vi "LCR_Main.vi"() -> ()   [LabVIEW 2021]
uses:
  GEN_States.ctl
  1375486a-d526-4950-a4e9-ede105372d37.vi
  Sources/Config_Cluster.ctl
  Sources/Data_Cluster.ctl
  <vilib>/Utility/config.llb/NI_LVConfig.lvlib
  Sources/Mode_Enum.ctl
  Sources/Measurement_Cluster.ctl
  <instrlib>/Hameg HM8118/Hameg HM8118.lvlib
  Sources/Plotting-Axis.ctl
panel:
  in  "Control Tab":enum32{"General", "Configs"}(tab)
  out "Capacitance":dbl
  in  "StopM_Button":bool
  in  "Log_Button":bool
  in  "Measure_Button":bool
  out "Globals":bool
  out "AH 2500A":bool
  out "Logging":bool
  out "Measuring":bool
  out "Magnetic Field":dbl
  out "Temperature":dbl
  in  "LoadConfig_Button":bool
  in  "ApplyConfig_Button":bool
  in  "Measure rate (1/s)":i32
  in  "SaveConfig_Button":bool
  in  "Default Measurement Profile":path
  in  "Retry_Button":bool
  in  "Restart on Load":bool
  in  "Config Path (Blank is default)":path
  in  "LCR VISA COM":refnum<visa-resource-name>
  in  "Global Temp VAR":refnum<k21>
  in  "Global Mag VAR":refnum<k21>
  in  "Logging Path":path
  in  "Display Tab":enum32{"Program Monitor", "Test Plot"}(tab)
  out "Status":string
  in  "Clear_Button":bool
  in  "Y-Axis":T1
  in  "X-Axis":T1
  out "Test Graph":cluster{"X":dbl, "Y":dbl}[](graph)
  in  "Max Elements":i32=5000
  in  "Exit_Button":bool
  # "Instrument Settings"
  # "Global Var. Settings"
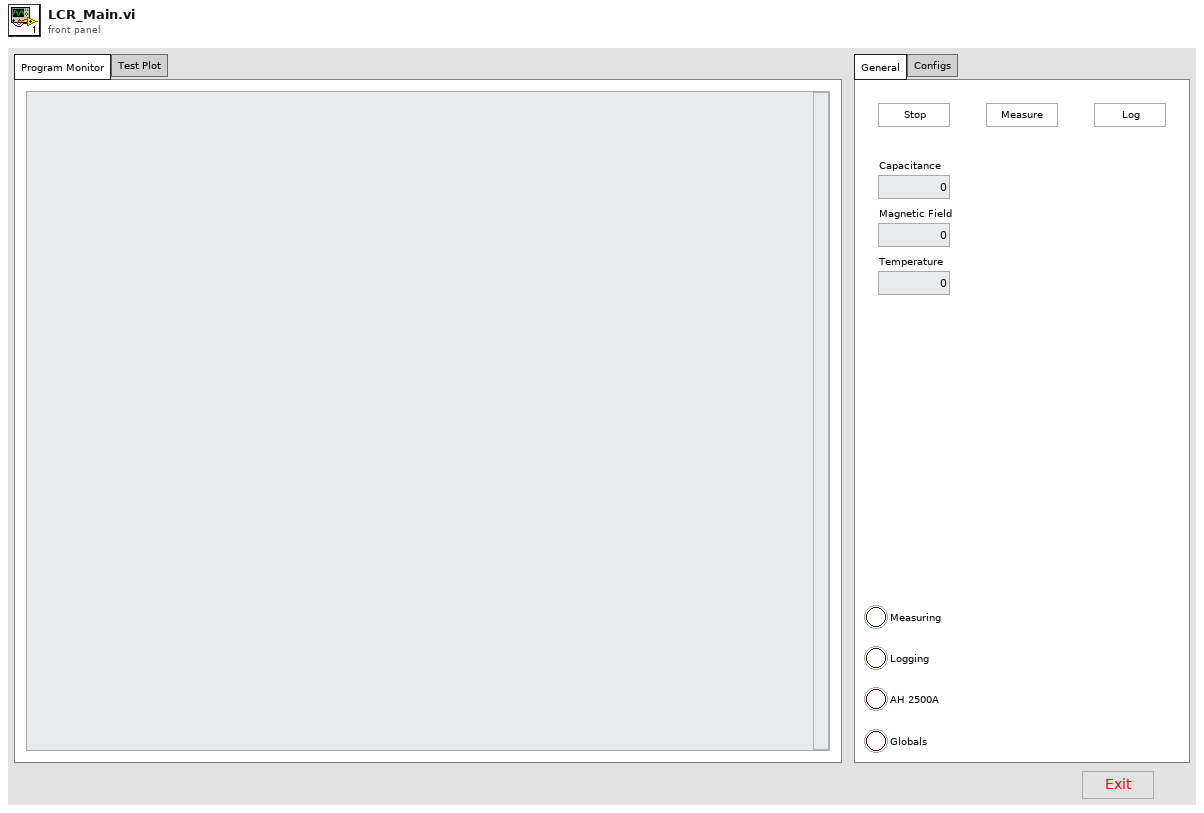
[diagram p1: front panel]
types:
  T1 = typedef "Plotting-Axis.ctl" = enum16{"Time", "Temperature", "MagneticField", "Primary", "Secondary"}
  T2 = typedef "GEN_States.ctl" = enum16{"ClearBuffers", "SwitchToMeas", "SwitchToLog", "SwitchToOff", "Disconnect", "ApplyConfig", "ExitSafe", "RefreshPlotMUnits", "UpdatePlots", "RefreshMUnits", "ChangeOperation", "Read/WriteAll", "RetryComs", "SendProfile", "InitGUI", "RefreshGUI", "ComsFail", "SaveConfig", "Idle", "ProgInit"}
  T3 = typedef "Data_Cluster.ctl" = cluster{"Value":dbl, "GUI Data Cluster":cluster{"Numeric":dbl}, "Timing":cluster{"Last Operation":dbl}, "Measurements":T4[]}
  T4 = typedef "Measurement_Cluster.ctl" = cluster{"Time Stamp":timestamp, "Cap":dbl, "Temperature":dbl, "MagneticField":dbl}
  T5 = typedef "Config_Cluster.ctl" = cluster{"General":cluster{"Config.ini":path, "Default Logging Path":path}, "Hardware":cluster{"AHC VISA COM":refnum<visa-resource-name>, "Measure Rate (1/s)":i32, "Global T VAR":refnum<k21>, "Global B VAR":refnum<k21>}, "Operation":cluster{"Operation Mode":T6, "Status":string, "NewLog?":bool}}
  T6 = typedef "Mode_Enum.ctl" = enum16{"Logging", "Idle-Off", "Idle"}
  T7 = enum8{"Enabled", "Disabled", "Disabled and Grayed Out"}
  T8 = typedef "NI_LVConfig.lvlib/Config Data RefNum.ctl" = refnum<k1>
  T9 = cluster{"Logging Path":path, "LCR VISA COM":refnum<visa-resource-name>, "Restart on Load":bool, "Default Measurement Profile":path, "Measure rate (1/s)":i32, "Global Temp VAR":refnum<k21>, "Global Mag VAR":refnum<k21>}
  T10 = cluster{"Primary Measurement":dbl, "Secondary Measurement":dbl, "T Var":dbl, "B Var":dbl}
  T11 = typedef "UnitEnum.ctl" = enum16{"L", "R", "C", "Z", "X", "Q", "Theta", "Y", "N", "M", "G", "B", "D"}
  T12 = typedef "GEN_States.ctl" = enum16{"ClearBuffers", "SwitchToMeas", "SwitchToLog", "SwitchToOff", "Disconnect", "ApplyConfig", "ExitSafe", "RefreshPlotMUnits", "UpdatePlots", "RefreshMUnits", "ChangeOperation", "Read/WriteAll", "RetryComs", "SendProfile", "InitGUI", "RefreshGUI", "ComsFail", "LoadProfile", "SaveProfile", "SaveConfig", "Idle", "ProgInit"}
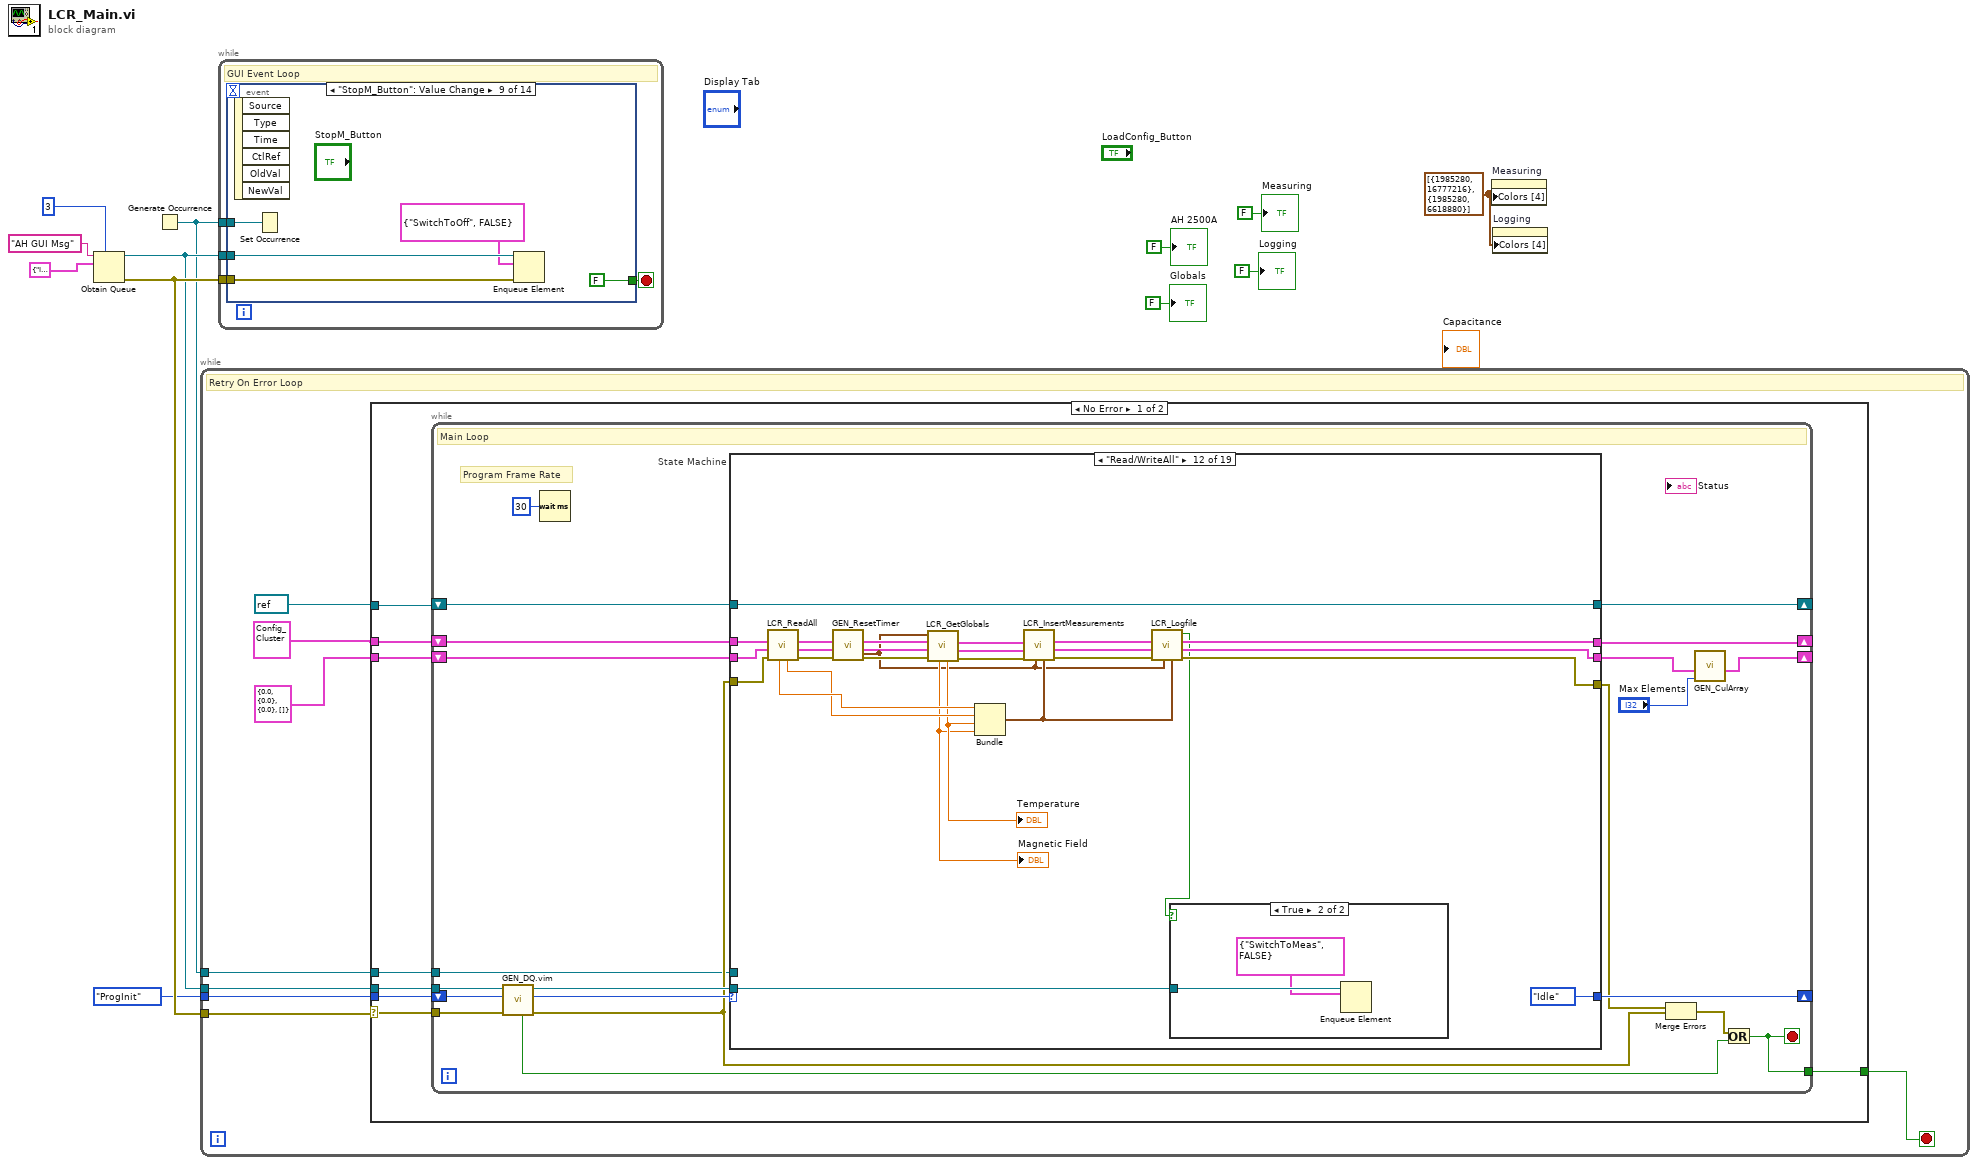
[diagram p0: block diagram]
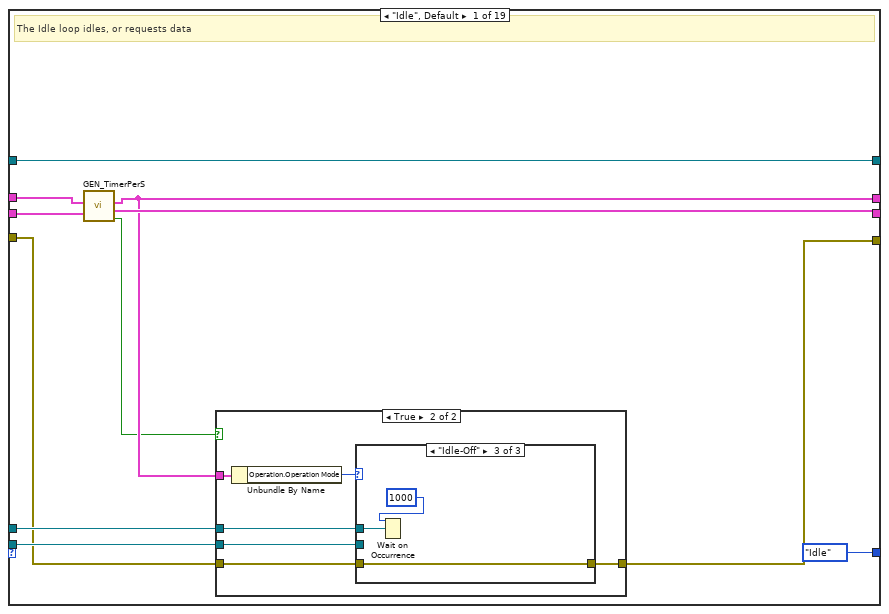
[diagram p2: hidden frame]
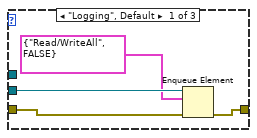
[diagram p4: hidden frame]
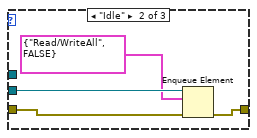
[diagram p5: hidden frame]
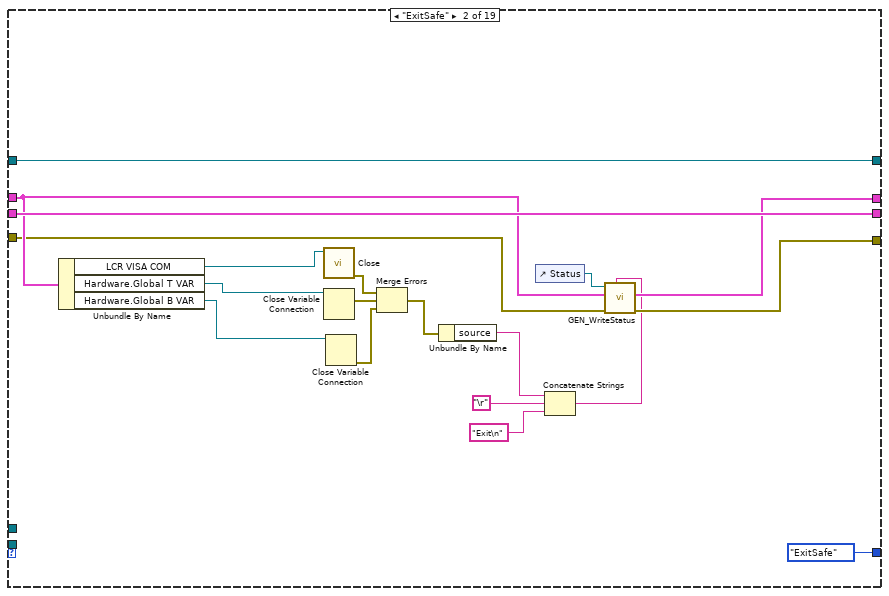
[diagram p6: hidden frame]
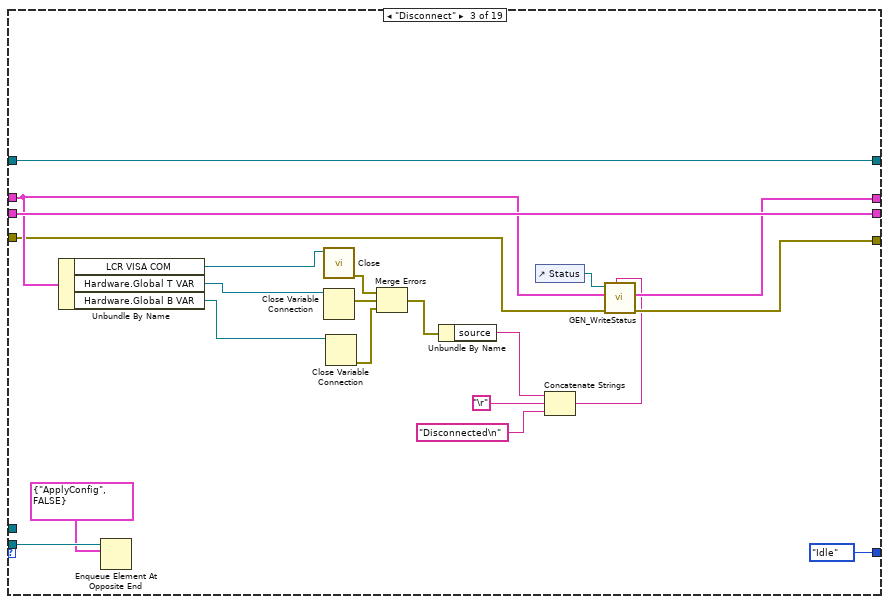
[diagram p7: hidden frame]
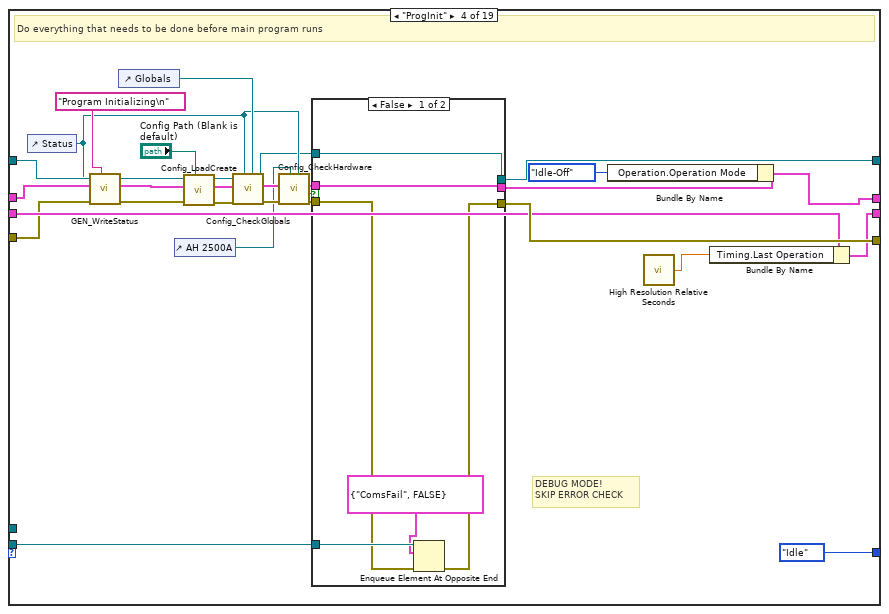
[diagram p8: hidden frame]
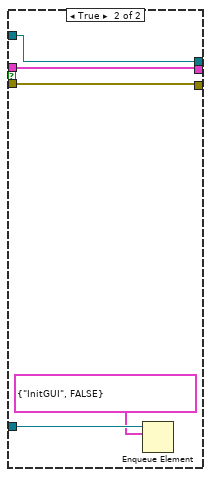
[diagram p9: hidden frame]
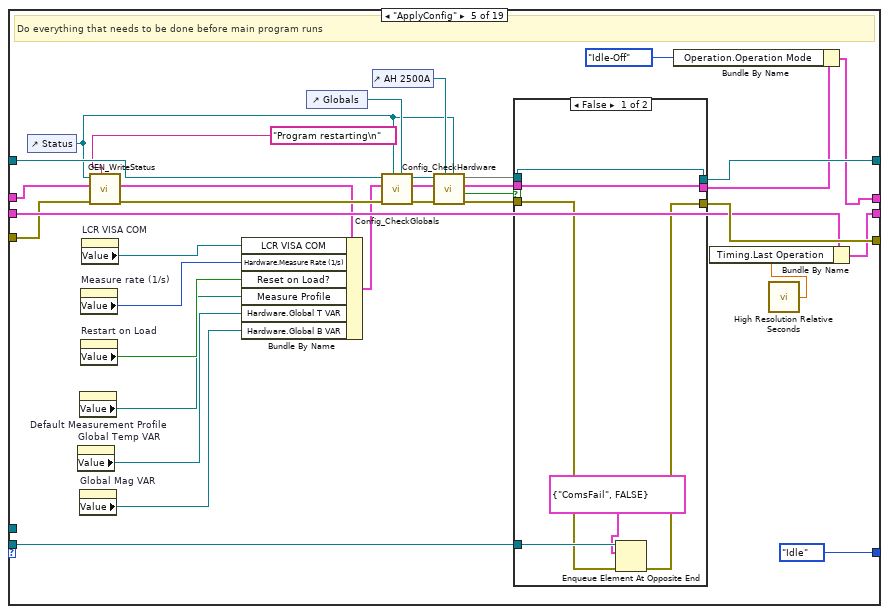
[diagram p10: hidden frame]
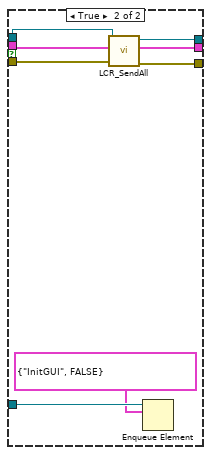
[diagram p11: hidden frame]
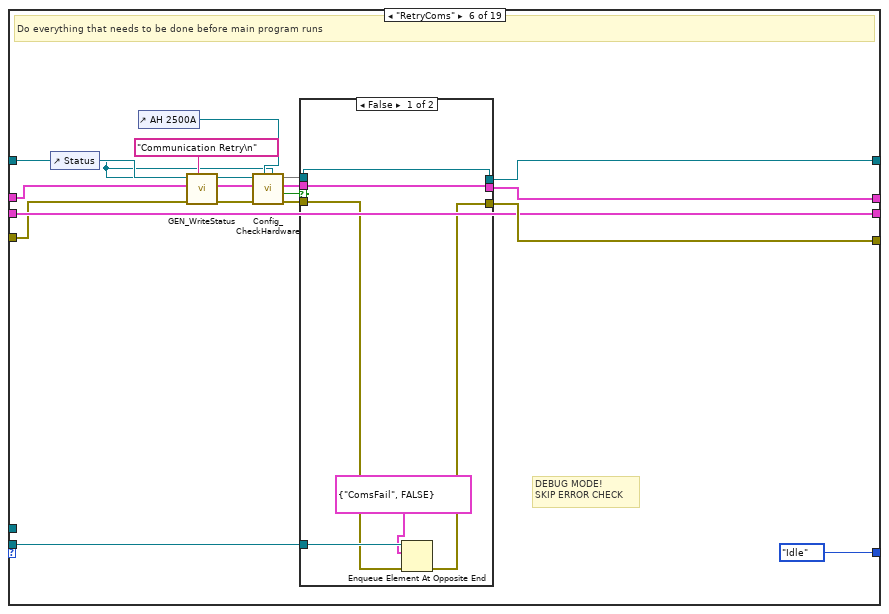
[diagram p12: hidden frame]
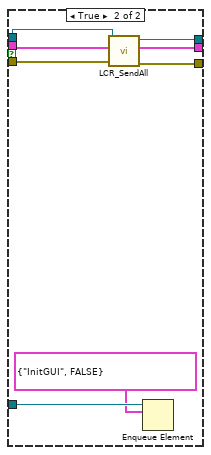
[diagram p13: hidden frame]
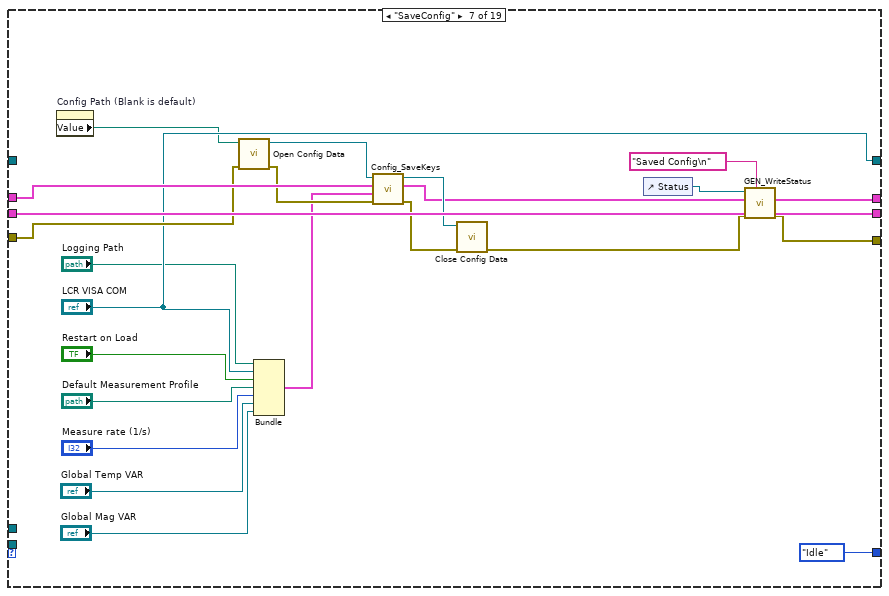
[diagram p14: hidden frame]
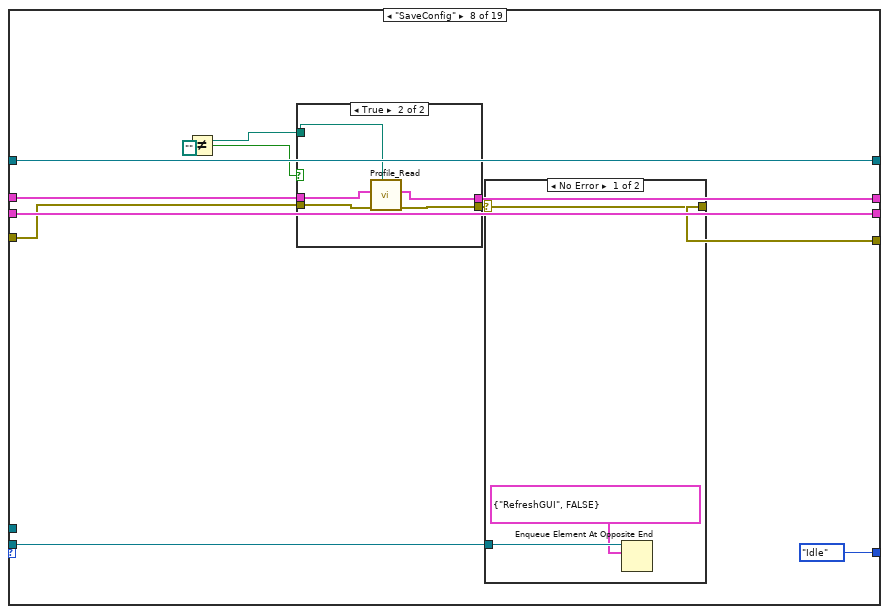
[diagram p15: hidden frame]
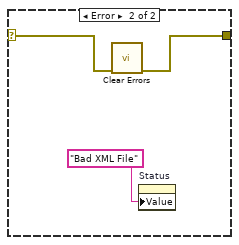
[diagram p16: hidden frame]
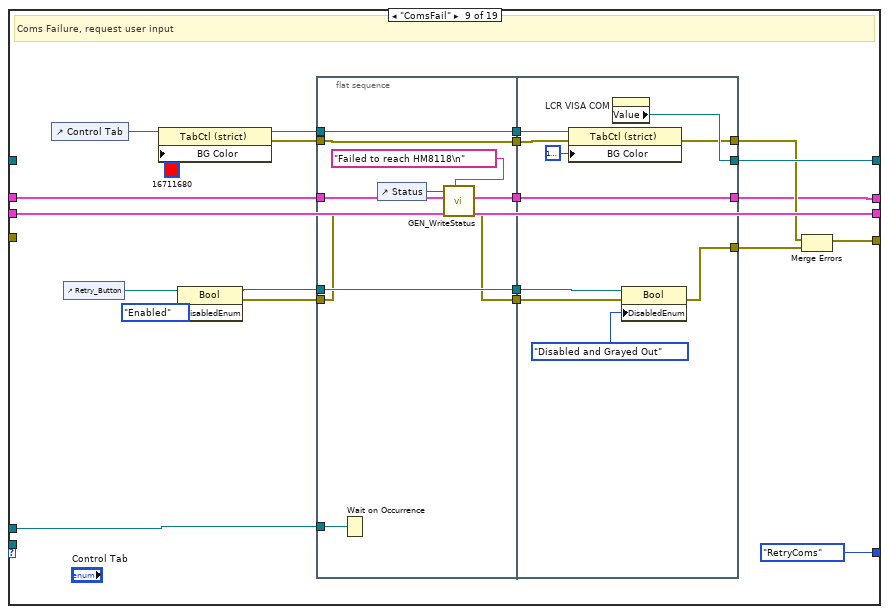
[diagram p18: hidden frame]
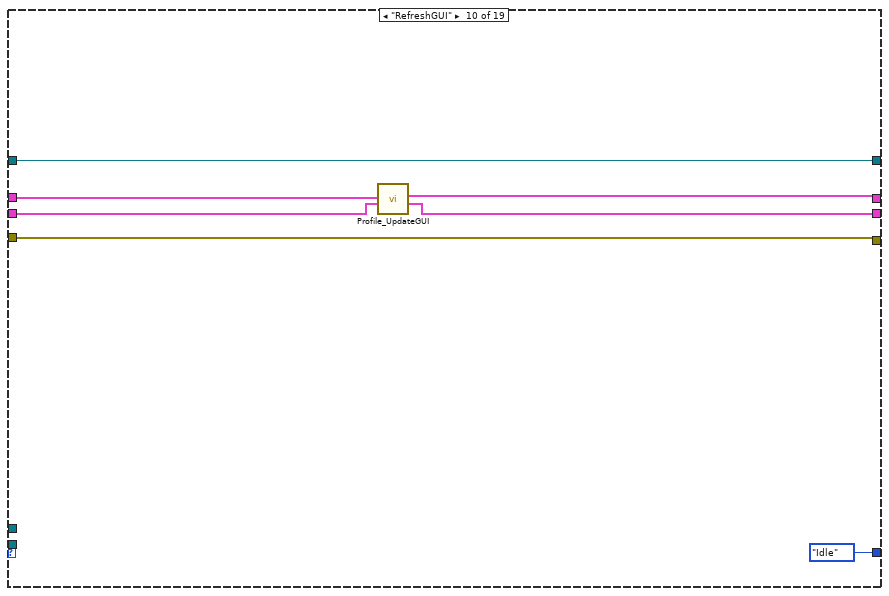
[diagram p19: hidden frame]
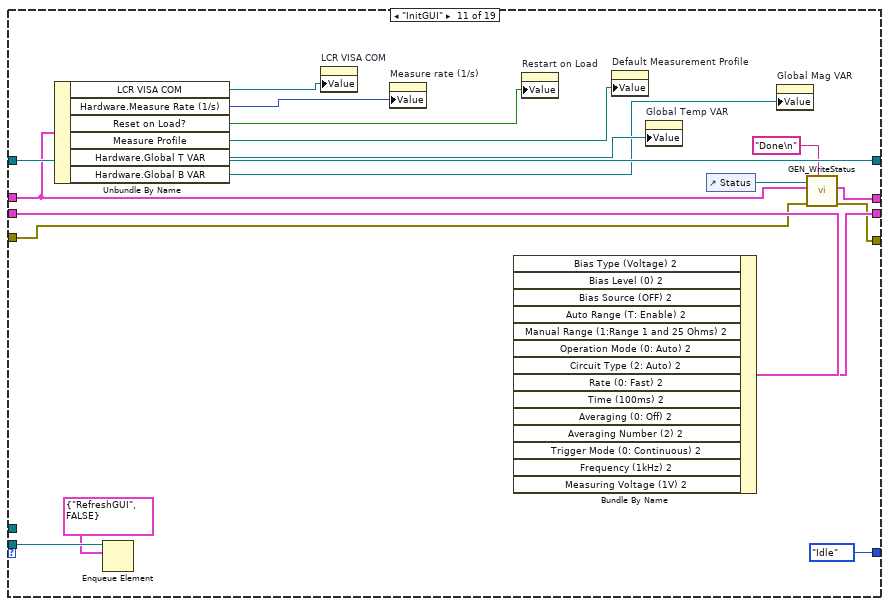
[diagram p20: hidden frame]
diagram:
  w1 = cluster{u32, u32}[] [{1985280, 16777216}, {1985280, 6618880}] ("Colors [4]")
  n1 = Obtain Queue(max queue size (-1, unlimited)=3, name (unnamed)="AH GUI Msg", element data type=cluster{T2, bool} {enum."Idle", TRUE}) -> (queue out=w8:refnum<queue>, error out=w9:errorcluster)  [unwired: 2 in, 1 out]
  n2 = Generate Occurrence() -> (w6:refnum<k4>)
  n3 = while {
    tunnel: w9 -> [w20]
    tunnel: w8 -> [w19]
    tunnel: GEN_States."ProgInit" ("State") -> [w18]
    tunnel: w6 -> [w13]
    stop <- w17 stop-if-true
    # "Retry On Error Loop"
    n4 = case shown="No Error" w20 {
      selector: w20 -> [w28 _]
      tunnel: w19 -> [w27 _]
      tunnel: w18 -> [w26 _]
      tunnel: [w25 TRUE] -> w17
      tunnel: refnum<visa-resource-name> refnum ("LCR VISA COM") -> [w24 _]
      tunnel: T5 {"General"={"Config.ini"=path "", "Default Logging Path"=path ""}, "Hardware"={"AHC VISA COM"="", "Measure Rate (1/s)"=0, "Global T VAR"="", "Global B VAR"=""}, "Operation"={"Operation Mode"=enum."Logging", "Status"="", "NewLog?"=FALSE}} -> [w23 _]
      tunnel: T3 {"Value"=0.0, "GUI Data Cluster"={"Numeric"=0.0}, "Timing"={"Last Operation"=0.0}, "Measurements"=[]} -> [w22 _]
      tunnel: w13 -> [w21 _]
      frame No Error {
        n5 = while {
          tunnel: w28 -> [w48]
          tunnel: w27 -> [w47]
          shift-right: [w40] -> _
          shift-left: w26 -> [w46]
          tunnel: [w42] -> w25
          shift-right: [w39] -> _
          shift-left: w24 -> [w41]
          shift-right: [w36] -> _
          shift-left: w23 -> [w37]
          shift-right: [w30] -> _
          shift-left: w22 -> [w35]
          tunnel: w21 -> [w32]
          stop <- w42 stop-if-true
          # "Program Frame Rate"
          # "Main Loop"
          n6 = call "GEN_DQ.vim"("error in (no error)"=w48, "Variant"=w46, "queue In"=w47) -> ("error out"=w34:errorcluster, "Variant Out"=w45:T2, "queue out"=w38:refnum<queue>, "Exit?"=w43:bool)  [unwired: 5 in]
          n7 = Wait (ms)(milliseconds to wait=u32 30) -> ()  [unwired: 1 out]
          n8 = case "State Machine" shown="\"Read/WriteAll\"" w45 {
            tunnel: w41 -> [w60 w97 w118 w145 w190 w222 _ w272 _ w333 w366 w394 w413 w431 w457 w476 w487 w497 w503]
            tunnel: [GEN_States."Idle" ("State") GEN_States."ExitSafe" ("State") GEN_States."Idle" ("State") GEN_States."Idle" ("State") GEN_States."Idle" ("State") GEN_States."Idle" ("State") GEN_States."Idle" ("State") GEN_States."Idle" ("State") GEN_States."RetryComs" ("State") GEN_States."Idle" ("State") GEN_States."Idle" ("State") GEN_States."Idle" ("State") GEN_States."Idle" ("State") GEN_States."Idle" ("State") w443 GEN_States."Idle" ("State") GEN_States."Idle" ("State") GEN_States."Idle" ("State") GEN_States."Idle" ("State")] -> w40
            tunnel: [w60 w97 w118 w140 w184 w215 "LCR VISA COM" w272 w300 w333 w366 w394 w413 w431 w457 w476 w487 w497 w503] -> w39
            tunnel: w38 -> [w57 _ w100 w139 w183 w214 _ w261 _ _ w362 w367 _ _ _ _ _ _ _]
            tunnel: w37 -> [w54 w90 w112 w131 w175 w212 w255 w268 w288 w328 w342 w393 w411 w429 w455 w477 w486 w494 w502]
            tunnel: [w51 w89 w111 w132 w176 w216 w245 w267 w287 w330 w341 w388 w408 w426 w444 w474 w486 w494 w502] -> w36
            tunnel: w35 -> [w53 w96 w117 w138 w182 w213 w260 w271 w302 w331 w365 w385 w412 w430 w456 w475 w482 w495 w500]
            tunnel: [w52 w96 w117 w137 w181 w213 w260 w271 w302 w329 w364 w382 w412 w430 w456 w475 w481 w495 w499] -> w31
            tunnel: w34 -> [w56 w88 w110 w129 w174 w209 w254 w269 _ w332 w339 w392 w403 w421 w449 w473 w480 w493 w501]
            tunnel: [w55 w87 w109 w141 w185 w217 w241 w262 w291 w332 w338 w389 w402 w420 w448 w468 w480 w493 w501] -> w33
            tunnel: w32 -> [w58 _ _ _ _ _ _ _ w301 _ _ _ _ _ _ _ _ _ _]
            frame "Idle", Default {
              # "The Idle loop idles, or requests data"
              n9 = call "GEN_TimerPerS.vi"("Data_In"=w53, "Config_In"=w54) -> ("Time"=w50:bool, "Data_In 2"=w52:T3, "Config_In 2"=w51:T5)  [unwired: 7 in]
              n10 = case shown="True" w50 {
                tunnel: w58 -> [_ w66]
                tunnel: w57 -> [_ w65]
                tunnel: w56 -> [w61 w64]
                tunnel: [w61 w63] -> w55
                tunnel: w51 -> [_ w62]
                frame False {
                }
                frame True {
                  n11 = Unbundle By Name(w62) -> ("Operation.Operation Mode"=w67:T6)
                  n12 = case shown="\"Idle-Off\"" w67 {
                    tunnel: w66 -> [_ _ w78]
                    tunnel: w65 -> [w71 w75 _]
                    tunnel: w64 -> [w70 w74 w77]
                    tunnel: [w68 w72 w77] -> w63
                    frame "Logging", Default {
                      n13 = Enqueue Element(queue=w71, element=cluster{T2, bool} {enum."Read/WriteAll", FALSE}, error in (no error)=w70) -> (error out=w68:errorcluster)  [unwired: 1 in, 2 out]
                    }
                    frame "Idle" {
                      n14 = Enqueue Element(queue=w75, element=cluster{T2, bool} {enum."Read/WriteAll", FALSE}, error in (no error)=w74) -> (error out=w72:errorcluster)  [unwired: 1 in, 2 out]
                    }
                    frame "Idle-Off" {
                      n15 = Wait on Occurrence(2:w78, 3:1000 ("ms timeout (-1)")) -> ()  [unwired: 1 in, 1 out]
                    }
                  }
                }
              }
            }
            frame "ExitSafe" {
              n16 = Unbundle By Name(w90) -> ("LCR VISA COM"=w94:refnum<visa-resource-name>, "Hardware.Global T VAR"=w93:refnum<k21>, "Hardware.Global B VAR"=w92:refnum<k21>)
              n17 = call <instrlib>:"Close.vi"("VISA resource name"=w94) -> ("error out"=w84:errorcluster)  [unwired: 10 in]
              n18 = Close Variable Connection(11:w93) -> (0:w85:errorcluster)  [unwired: 1 in]
              n19 = Close Variable Connection(11:w92) -> (0:w86:errorcluster)  [unwired: 1 in]
              n20 = Merge Errors(w84, w85, w86) -> (w83:errorcluster)
              n21 = Unbundle By Name(w83) -> ("source"=w81:string)
              n22 = control-ref of="Status"() -> (w91:refnum<vi>)
              n23 = Concatenate Strings(w81, "\r", "Exit\n" ("string")) -> (w82:string)
              n24 = call "GEN_WriteStatus.vi"("Input String"=w82, "error in (no error)"=w88, "Config_Cluster"=w90, "Status Ref"=w91) -> ("error out"=w87:errorcluster, "Config_Cluster Out"=w89:T5)  [unwired: 6 in]
            }
            frame "Disconnect" {
              n25 = Unbundle By Name(w112) -> ("LCR VISA COM"=w116:refnum<visa-resource-name>, "Hardware.Global T VAR"=w115:refnum<k21>, "Hardware.Global B VAR"=w114:refnum<k21>)
              n26 = Enqueue Element At Opposite End(queue=w100, element=cluster{T2, bool} {enum."ApplyConfig", FALSE}) -> ()  [unwired: 2 in, 3 out]
              n27 = call <instrlib>:"Close.vi"("VISA resource name"=w116) -> ("error out"=w106:errorcluster)  [unwired: 10 in]
              n28 = Close Variable Connection(11:w115) -> (0:w107:errorcluster)  [unwired: 1 in]
              n29 = Close Variable Connection(11:w114) -> (0:w108:errorcluster)  [unwired: 1 in]
              n30 = Merge Errors(w106, w107, w108) -> (w105:errorcluster)
              n31 = Unbundle By Name(w105) -> ("source"=w103:string)
              n32 = control-ref of="Status"() -> (w113:refnum<vi>)
              n33 = Concatenate Strings(w103, "\r", "Disconnected\n" ("string")) -> (w104:string)
              n34 = call "GEN_WriteStatus.vi"("Input String"=w104, "error in (no error)"=w110, "Config_Cluster"=w112, "Status Ref"=w113) -> ("error out"=w109:errorcluster, "Config_Cluster Out"=w111:T5)  [unwired: 6 in]
            }
            frame "ProgInit" {
              # "DEBUG MODE!\nSKIP ERROR CHECK"
              # "Do everything that needs to be done before main program runs"
              n35 = control-ref of="Status"() -> (w120:refnum<vi>)
              n36 = call "GEN_WriteStatus.vi"("Input String"="Program Initializing\n" ("Status"), "error in (no error)"=w129, "Config_Cluster"=w131, "Status Ref"=w120) -> ("error out"=w128:errorcluster, "Config_Cluster Out"=w130:T5)  [unwired: 6 in]
              n37 = control-ref of="Globals"() -> (w122:refnum<vi>)
              n38 = control-ref of="AH 2500A"() -> (w121:refnum<vi>)
              n39 = call "Config_LoadCreate.vi"("Config In"="Config Path (Blank is default)", "error In"=w128, "Configuration Cluster"=w130, "AH VISA COM"=w145) -> ("error out"=w124:errorcluster, "Configuration Cluster Out"=w125:T5, "AHC VISA COM Out"=w127:refnum<visa-resource-name>)  [unwired: 5 in]
              n40 = call "Config_CheckGlobals.vi"("GlobalsLED Ref"=w122, "Status Ref"=w120, "error in (no error)"=w124, "Config Cluster"=w125, "VISA resource name"=w127) -> ("error out"=w123:errorcluster, "Config Cluster Out"=w126:T5, "VISA resource name out"=w119:refnum<visa-resource-name>)  [unwired: 4 in]
              n41 = call "Config_CheckHardware.vi"("Status Ref"=w120, "HM 8119"=w121, "error in (no error)"=w123, "Config Cluster"=w126) -> ("error out"=w143:errorcluster, "Connected?"=w144:bool, "Config Cluster Out"=w142:T5)  [unwired: 5 in]
              n42 = case shown="False" w144 {
                tunnel: w143 -> [w149 w157]
                tunnel: w142 -> [w152 w158]
                tunnel: w119 -> [w153 w154]
                tunnel: [w153 w154] -> w140
                tunnel: [w152 w158] -> w135
                tunnel: [w148 w157] -> w141
                tunnel: w139 -> [w151 w156]
                frame False {
                  n43 = Enqueue Element At Opposite End(queue=w151, element=cluster{T2, bool} {enum."ComsFail", FALSE}, error in (no error)=w149) -> (error out=w148:errorcluster)  [unwired: 1 in, 2 out]
                }
                frame True {
                  n44 = Enqueue Element(queue=w156, element=cluster{T2, bool} {enum."InitGUI", FALSE}) -> ()  [unwired: 2 in, 3 out]
                }
              }
              n45 = Bundle By Name(cluster=w135, "Operation.Operation Mode"=Mode_Enum."Idle-Off") -> (w132:T5)
              n46 = call <vilib>:"High Resolution Relative Seconds.vi"() -> ("relative seconds"=w136:dbl)
              n47 = Bundle By Name(cluster=w138, "Timing.Last Operation"=w136) -> (w137:T3)
            }
            frame "ApplyConfig" {
              # "Do everything that needs to be done before main program runs"
              n48 = control-ref of="Status"() -> (w159:refnum<vi>)
              n49 = property on="Global Temp VAR" class="Variable (strict)"() -> ("Value"=w163:refnum<k21>)  [unwired: 2 in, 2 out]
              n50 = property on="Default Measurement Profile" class="Path"() -> ("Value"=w164:path)  [unwired: 2 in, 2 out]
              n51 = property on="Global Mag VAR" class="Variable (strict)"() -> ("Value"=w162:refnum<k21>)  [unwired: 2 in, 2 out]
              n52 = property on="Measure rate (1/s)" class="DigNum (strict)"() -> ("Value"=w166:i32)  [unwired: 2 in, 2 out]
              n53 = property on="Restart on Load" class="Bool (strict)"() -> ("Value"=w165:bool)  [unwired: 2 in, 2 out]
              n54 = property on="LCR VISA COM" class="VISAName"() -> ("Value"=w167:refnum<visa-resource-name>)  [unwired: 2 in, 2 out]
              n55 = call "GEN_WriteStatus.vi"("Input String"="Program restarting\n" ("Status"), "error in (no error)"=w174, "Config_Cluster"=w175, "Status Ref"=w159) -> ("error out"=w173:errorcluster, "Config_Cluster Out"=w169:T5)  [unwired: 6 in]
              n56 = Bundle By Name(cluster=w169, "LCR VISA COM"=w167, "Hardware.Measure Rate (1/s)"=w166, "Reset on Load?"=w165, "Measure Profile"=w164, "Hardware.Global T VAR"=w163, "Hardware.Global B VAR"=w162) -> (w168:T5)
              n57 = control-ref of="Globals"() -> (w161:refnum<vi>)
              n58 = control-ref of="AH 2500A"() -> (w160:refnum<vi>)
              n59 = call "Config_CheckGlobals.vi"("GlobalsLED Ref"=w161, "Status Ref"=w159, "error in (no error)"=w173, "Config Cluster"=w168, "VISA resource name"=w190) -> ("error out"=w170:errorcluster, "Config Cluster Out"=w171:T5, "VISA resource name out"=w172:refnum<visa-resource-name>)  [unwired: 4 in]
              n60 = call "Config_CheckHardware.vi"("Status Ref"=w159, "HM 8119"=w160, "error in (no error)"=w170, "Config Cluster"=w171, 11:w172) -> ("error out"=w188:errorcluster, "Connected?"=w189:bool, "Config Cluster Out"=w187:T5, 3:w186)  [unwired: 3 in]
              n61 = case shown="False" w189 {
                tunnel: w188 -> [w193 w203]
                tunnel: w187 -> [w196 w204]
                tunnel: w186 -> [w197 w205]
                tunnel: [w197 w202] -> w184
                tunnel: [w196 w201] -> w179
                tunnel: [w192 w200] -> w185
                tunnel: w183 -> [w195 w199]
                frame False {
                  n62 = Enqueue Element At Opposite End(queue=w195, element=cluster{T2, bool} {enum."ComsFail", FALSE}, error in (no error)=w193) -> (error out=w192:errorcluster)  [unwired: 1 in, 2 out]
                }
                frame True {
                  n63 = call "LCR_SendAll.vi"("error in (no error)"=w203, "Configuration Cluster"=w204, "VISA resource name"=w205) -> ("error out"=w200:errorcluster, "Configuration Cluster Out"=w201:T5, "VISA resource name out"=w202:refnum<visa-resource-name>)  [unwired: 6 in]
                  n64 = Enqueue Element(queue=w199, element=cluster{T2, bool} {enum."InitGUI", FALSE}) -> ()  [unwired: 2 in, 3 out]
                }
              }
              n65 = Bundle By Name(cluster=w179, "Operation.Operation Mode"=Mode_Enum."Idle-Off") -> (w176:T5)
              n66 = call <vilib>:"High Resolution Relative Seconds.vi"() -> ("relative seconds"=w180:dbl)
              n67 = Bundle By Name(cluster=w182, "Timing.Last Operation"=w180) -> (w181:T3)
            }
            frame "RetryComs" {
              # "DEBUG MODE!\nSKIP ERROR CHECK"
              # "Do everything that needs to be done before main program runs"
              n68 = control-ref of="Status"() -> (w206:refnum<vi>)
              n69 = control-ref of="AH 2500A"() -> (w207:refnum<vi>)
              n70 = call "GEN_WriteStatus.vi"("Input String"="Communication Retry\n", "error in (no error)"=w209, "Config_Cluster"=w212, "Status Ref"=w206) -> ("error out"=w208:errorcluster, "Config_Cluster Out"=w211:T5)  [unwired: 6 in]
              n71 = call "Config_CheckHardware.vi"("Status Ref"=w206, "HM 8119"=w207, "error in (no error)"=w208, "Config Cluster"=w211, 11:w222) -> ("error out"=w220:errorcluster, "Connected?"=w221:bool, "Config Cluster Out"=w219:T5, 3:w218)  [unwired: 3 in]
              n72 = case shown="False" w221 {
                tunnel: w220 -> [w225 w235]
                tunnel: w219 -> [w228 w236]
                tunnel: w218 -> [w229 w237]
                tunnel: [w229 w234] -> w215
                tunnel: [w228 w233] -> w216
                tunnel: [w224 w232] -> w217
                tunnel: w214 -> [w227 w231]
                frame False {
                  n73 = Enqueue Element At Opposite End(queue=w227, element=cluster{T2, bool} {enum."ComsFail", FALSE}, error in (no error)=w225) -> (error out=w224:errorcluster)  [unwired: 1 in, 2 out]
                }
                frame True {
                  n74 = call "LCR_SendAll.vi"("error in (no error)"=w235, "Configuration Cluster"=w236, "VISA resource name"=w237) -> ("error out"=w232:errorcluster, "Configuration Cluster Out"=w233:T5, "VISA resource name out"=w234:refnum<visa-resource-name>)  [unwired: 6 in]
                  n75 = Enqueue Element(queue=w231, element=cluster{T2, bool} {enum."InitGUI", FALSE}) -> ()  [unwired: 2 in, 3 out]
                }
              }
            }
            frame "SaveConfig" {
              n76 = property on="Config Path (Blank is default)" class="Path"() -> ("Value"=w248:path)  [unwired: 2 in, 2 out]
              n77 = call <vilib>:"Open Config Data.vi"("error in (no error)"=w254, "configuration file path"=w248) -> ("error out"=w253:errorcluster, "refnum"=w252:T8)  [unwired: 7 in, 1 out]
              n78 = Bundle("Logging Path"="Logging Path", "LCR VISA COM"="LCR VISA COM", "Restart on Load"="Restart on Load", "Default Measurement Profile"="Default Measurement Profile", "Measure rate (1/s)"="Measure rate (1/s)", "Global Temp VAR"="Global Temp VAR", "Global Mag VAR"="Global Mag VAR") -> (w238:T9)  [unwired: 1 in]
              n79 = call "Config_SaveKeys.vi"("error in (no error)"=w253, "Settings In"=w238, "Configuration Cluster"=w255, "Config In"=w252) -> ("error out"=w250:errorcluster, "output cluster"=w246:T5, "refnum out"=w251:T8)  [unwired: 5 in]
              n80 = call <vilib>:"Close Config Data.vi"("error in (no error)"=w250, "refnum"=w251) -> ("error out"=w242:errorcluster)  [unwired: 8 in, 1 out]
              n81 = control-ref of="Status"() -> (w243:refnum<vi>)
              n82 = call "GEN_WriteStatus.vi"("Input String"="Saved Config\n", "error in (no error)"=w242, "Config_Cluster"=w246, "Status Ref"=w243) -> ("error out"=w241:errorcluster, "Config_Cluster Out"=w245:T5)  [unwired: 6 in]
            }
            frame "SaveConfig" {
              n83 = Not Equal?(x=w266, y=path "") -> (x != y?=w264:bool)
              n84 = case shown="True" w264 {
                tunnel: w269 -> [w279 w285]
                tunnel: w268 -> [w280 w284]
                tunnel: [_ w283] -> w266
                tunnel: [w279 w282] -> w263
                tunnel: [w280 w281] -> w267
                frame False {
                }
                frame True {
                  n85 = call "Profile_Read.vi"("Measurement Profile"=w283, "error in (no error)"=w285, "Configuration Cluster"=w284) -> ("error out"=w282:errorcluster, "Configuration Cluster Out"=w281:T5)  [unwired: 7 in]
                }
              }
              n86 = case shown="No Error" w263 {
                selector: w263 -> [w275 w278]
                tunnel: [w275 w277] -> w262
                tunnel: w261 -> [w274 _]
                frame No Error {
                  n87 = Enqueue Element At Opposite End(queue=w274, element=cluster{T2, bool} {enum."RefreshGUI", FALSE}) -> ()  [unwired: 2 in, 3 out]
                }
                frame Error {
                  n88 = call <vilib>:"Clear Errors.vi"("error in (no error)"=w278) -> ("error out"=w277:errorcluster)  [unwired: 5 in, 1 out]
                  n89 = property on="Status" class="Str"("Value"="Bad XML File" ("Status")) -> ()  [unwired: 2 in, 2 out]
                }
              }
            }
            frame "ComsFail" {
              # "Coms Failure, request user input"
              n90 = control-ref of="Control Tab"() -> (w307:refnum<vi>)
              n91 = control-ref of="Retry_Button"() -> (w306:refnum<vi>)
              n92 = property on="Property Node" class="TabCtl (strict)"(reference=w307, "BG Color"=u32 16711680 ("Colors:BG Color")) -> (reference out=w298:refnum<vi>, error out=w297:errorcluster)  [unwired: 1 in]
              n93 = property class="Bool"(reference=w306, "DisabledEnum"=T7."Enabled" ("Disabled")) -> (reference out=w294:refnum<vi>, error out=w293:errorcluster)  [unwired: 1 in]
              n94 = flat-sequence {
                tunnel: w301 -> [w317]
                tunnel: [w316] -> w299
                tunnel: w298 -> [w316]
                tunnel: w297 -> [w315]
                tunnel: [w315] -> w296
                tunnel: [w314] -> w295
                tunnel: w294 -> [w314]
                tunnel: w293 -> [w310]
                tunnel: [w309] -> w292
                tunnel: w288 -> [w313]
                tunnel: [w312] -> w286
                tunnel: [w327] -> w300
                tunnel: w299 -> [w326]
                tunnel: w296 -> [w325]
                tunnel: w295 -> [w324]
                tunnel: w292 -> [w323]
                tunnel: [w321] -> w290
                tunnel: [w320] -> w289
                tunnel: [w318] -> w287
                tunnel: w286 -> [w318]
                frame #0 {
                  n95 = Wait on Occurrence(2:w317) -> ()  [unwired: 2 in, 1 out]
                  n96 = control-ref of="Status"() -> (w308:refnum<vi>)
                  n97 = call "GEN_WriteStatus.vi"("Input String"="Failed to reach HM8118\n", "error in (no error)"=w310, "Config_Cluster"=w313, "Status Ref"=w308) -> ("error out"=w309:errorcluster, "Config_Cluster Out"=w312:T5)  [unwired: 6 in]
                }
                frame #1 {
                  n98 = property class="TabCtl (strict)"(reference=w326, error in=w325, "BG Color"=u32 16777226 ("Colors:BG Color")) -> (error out=w321:errorcluster)  [unwired: 1 out]
                  n99 = property on="LCR VISA COM" class="VISAName"() -> ("Value"=w327:refnum<visa-resource-name>)  [unwired: 2 in, 2 out]
                  n100 = property class="Bool"(reference=w324, error in=w323, "DisabledEnum"=T7."Disabled and Grayed Out" ("Disabled")) -> (error out=w320:errorcluster)  [unwired: 1 out]
                }
              }
              n101 = Merge Errors(w290, w289) -> (w291:errorcluster)
            }
            frame "RefreshGUI" {
              n102 = call "Profile_UpdateGUI.vi"("Data Cluster"=w331, "Configuration Cluster"=w328) -> ("Data Cluster Out"=w329:T3, "Configuration Cluster Out"=w330:T5)  [unwired: 8 in]
            }
            frame "InitGUI" {
              n103 = Unbundle By Name(w342) -> ("LCR VISA COM"=w346:refnum<visa-resource-name>, "Hardware.Measure Rate (1/s)"=w345:i32, "Reset on Load?"=w344:bool, "Measure Profile"=w343:path, "Hardware.Global T VAR"=w336:refnum<k21>, "Hardware.Global B VAR"=w335:refnum<k21>)
              n104 = Enqueue Element(queue=w362, element=cluster{T2, bool} {enum."RefreshGUI", FALSE}) -> ()  [unwired: 2 in, 3 out]
              n105 = property on="LCR VISA COM" class="VISAName"("Value"=w346) -> ()  [unwired: 2 in, 2 out]
              n106 = property on="Measure rate (1/s)" class="DigNum (strict)"("Value"=w345) -> ()  [unwired: 2 in, 2 out]
              n107 = Bundle By Name(cluster=w365) -> (w364:T3, "Bias Type (Voltage) 2"=w360:refnum<vi>, "Bias Level (0) 2"=w359:refnum<vi>, "Bias Source (OFF) 2"=w358:refnum<vi>, "Auto Range (T: Enable) 2"=w357:refnum<vi>, "Manual Range (1:Range 1 and 25 Ohms) 2"=w356:refnum<vi>, "Operation Mode (0: Auto) 2"=w355:refnum<vi>, "Circuit Type (2: Auto) 2"=w354:refnum<vi>, "Rate (0: Fast) 2"=w353:refnum<vi>, "Time (100ms) 2"=w351:refnum<vi>, "Averaging (0: Off) 2"=w352:refnum<vi>, "Averaging Number (2) 2"=w350:refnum<vi>, "Trigger Mode (0: Continuous) 2"=w349:refnum<vi>, "Frequency (1kHz) 2"=w348:refnum<vi>, "Measuring Voltage (1V) 2"=w347:refnum<vi>)
              n108 = property on="Restart on Load" class="Bool (strict)"("Value"=w344) -> ()  [unwired: 2 in, 2 out]
              n109 = property on="Default Measurement Profile" class="Path"("Value"=w343) -> ()  [unwired: 2 in, 2 out]
              n110 = property on="Global Temp VAR" class="Variable (strict)"("Value"=w336) -> ()  [unwired: 2 in, 2 out]
              n111 = control-ref of="Status"() -> (w337:refnum<vi>)
              n112 = property on="Global Mag VAR" class="Variable (strict)"("Value"=w335) -> ()  [unwired: 2 in, 2 out]
              n113 = call "GEN_WriteStatus.vi"("Input String"="Done\n", "error in (no error)"=w339, "Config_Cluster"=w342, "Status Ref"=w337) -> ("error out"=w338:errorcluster, "Config_Cluster Out"=w341:T5)  [unwired: 6 in]
            }
            frame "Read/WriteAll" {
              n114 = call "LCR_ReadAll.vi"("error in (no error)"=w392, "Data_In"=w385, "Configuration Cluster"=w393) -> ("error out"=w391:errorcluster, "Data_Out"=w384:T3, "Configuration Cluster 2"=w387:T5, "Secondary Measurement"=w380:dbl, "Primary Measurement"=w381:dbl)  [unwired: 4 in]
              n115 = call "GEN_ResetTimer.vi"("error in (no error)"=w391, "Data_In"=w384, "Cluster IN"=w387) -> ("error out"=w376:errorcluster, "Data_In 2"=w377:T3, "Cluster OUT"=w378:T5, "TimeStamp"=w370:timestamp)  [unwired: 5 in]
              n116 = call "LCR_GetGlobals.vi"("error in (no error)"=w376, "Data_In"=w377, "Cluster IN"=w378, "Start Stamp"=w370) -> ("error out"=w373:errorcluster, "Data_Out"=w374:T3, "Cluster OUT"=w375:T5, "T Var"=w372:dbl, "B Var"=w371:dbl)  [unwired: 1 in, 2 out]
              "Temperature" <- w372
              "Magnetic Field" <- w371
              n117 = Bundle("Primary Measurement"=w381, "Secondary Measurement"=w380, "T Var"=w372, "B Var"=w371) -> (w379:T10)  [unwired: 1 in]
              n118 = call "LCR_InsertMeasurements.vi"("Data Cluster"=w379, "TimeStamp"=w370, "error in (no error)"=w373, "Data_IN"=w374, "Cluster IN"=w375) -> ("error out"=w369:errorcluster, "Data_OUT"=w383:T3, "Cluster OUT"=w386:T5)  [unwired: 4 in]
              n119 = call "LCR_Logfile.vi"("Data Cluster"=w379, "Time Stamp"=w370, "error in"=w369, "Data_In"=w383, "Config_In"=w386) -> ("error out"=w389:errorcluster, "Data_Out"=w382:T3, "Config_Out"=w388:T5, "File Failure"=w368:bool)  [unwired: 3 in]
              n120 = case shown="True" w368 {
                tunnel: w367 -> [w396 w398]
                frame False {
                  n121 = Enqueue Element(queue=w396, element=cluster{T2, bool} {enum."UpdatePlots", FALSE}) -> ()  [unwired: 2 in, 3 out]
                }
                frame True {
                  n122 = Enqueue Element(queue=w398, element=cluster{T2, bool} {enum."SwitchToMeas", FALSE}) -> ()  [unwired: 2 in, 3 out]
                }
              }
            }
            frame "SwitchToOff" {
              w407 = Mode_Enum."Idle-Off" ("Operation.Operation Mode")
              n123 = Bundle By Name(cluster=w411, "Operation.Operation Mode"=w407) -> (w409:T5)
              n124 = case shown="\"Logging\", Default" w407 {
                tunnel: ["Measure and logging\n" "Off\n" "Measure only\n"] -> w406
                frame "Logging", Default {
                }
                frame "Idle-Off" {
                }
                frame "Idle" {
                }
              }
              n125 = control-ref of="Status"() -> (w401:refnum<vi>)
              n126 = Concatenate Strings("Changed Mode to: " ("string"), w406) -> (w404:string)
              n127 = call "GEN_WriteStatus.vi"("Input String"=w404, "error in (no error)"=w403, "Config_Cluster"=w409, "Status Ref"=w401) -> ("error out"=w402:errorcluster, "Config_Cluster Out"=w408:T5)  [unwired: 6 in]
              n128 = property on="Measuring" class="Bool (strict)"("Value"=FALSE ("Measuring")) -> ()  [unwired: 2 in, 2 out]
              n129 = property on="Logging" class="Bool (strict)"("Value"=FALSE ("Logging")) -> ()  [unwired: 2 in, 2 out]
            }
            frame "SwitchToMeas" {
              w425 = Mode_Enum."Idle" ("Operation.Operation Mode")
              n130 = Bundle By Name(cluster=w429, "Operation.Operation Mode"=w425) -> (w427:T5)
              n131 = case shown="\"Idle\"" w425 {
                tunnel: ["Measure and logging\n" "Off\n" "Measure only\n"] -> w424
                frame "Logging", Default {
                }
                frame "Idle-Off" {
                }
                frame "Idle" {
                }
              }
              n132 = control-ref of="Status"() -> (w419:refnum<vi>)
              n133 = Concatenate Strings("Changed Mode to: " ("string"), w424) -> (w422:string)
              n134 = call "GEN_WriteStatus.vi"("Input String"=w422, "error in (no error)"=w421, "Config_Cluster"=w427, "Status Ref"=w419) -> ("error out"=w420:errorcluster, "Config_Cluster Out"=w426:T5)  [unwired: 6 in]
              n135 = property on="Measuring" class="Bool (strict)"("Value"=TRUE ("Measuring")) -> ()  [unwired: 2 in, 2 out]
              n136 = property on="Logging" class="Bool (strict)"("Value"=FALSE ("Logging")) -> ()  [unwired: 2 in, 2 out]
            }
            frame "SwitchToLog" {
              w453 = Mode_Enum."Logging" ("Operation.Operation Mode")
              n137 = call "File Dialog"("prompt"="Where do you want to log measurements?", "default name"="LogFile.csv", "pattern (all files)"="*.csv", "pattern label"="CSV file") -> ("selected path"=w442:path, "cancelled"=w446:bool)  [unwired: 8 in, 2 out]
              n138 = Bundle By Name(cluster=w455, "Operation.Operation Mode"=w453, "Operation.NewLog?"=TRUE) -> (w454:T5)
              n139 = case shown="\"Logging\", Default" w453 {
                tunnel: ["Measure and logging\n" "Off\n" "Measure only\n"] -> w452
                frame "Logging", Default {
                }
                frame "Idle-Off" {
                }
                frame "Idle" {
                }
              }
              n140 = control-ref of="Status"() -> (w447:refnum<vi>)
              n141 = Concatenate Strings("Changed Mode to: " ("string"), w452) -> (w450:string)
              n142 = property on="Logging" class="Bool (strict)"("Value"=TRUE ("Logging")) -> ()  [unwired: 2 in, 2 out]
              n143 = property on="Measuring" class="Bool (strict)"("Value"=TRUE ("Measuring")) -> ()  [unwired: 2 in, 2 out]
              n144 = call "GEN_WriteStatus.vi"("Input String"=w450, "error in (no error)"=w449, "Config_Cluster"=w454, "Status Ref"=w447) -> ("error out"=w448:errorcluster, "Config_Cluster Out"=w445:T5)  [unwired: 6 in]
              n145 = case shown="False" w446 {
                tunnel: w445 -> [w460 w462]
                tunnel: [w459 w462] -> w444
                tunnel: [GEN_States."RefreshMUnits" ("State") GEN_States."SwitchToMeas" ("State")] -> w443
                tunnel: w442 -> [w458 _]
                frame False {
                  n146 = Bundle By Name(cluster=w460, "General.Default Logging Path"=w458) -> (w459:T5)
                }
                frame True {
                }
              }
            }
            frame "RefreshMUnits" {
              n147 = call "LCR_ReadMType.vi"("error in (no error)"=w473, "Configuration Cluster"=w477) -> ("error out"=w468:errorcluster, "Configuration Cluster Out"=w474:T5, "Secondary Unit"=w471:T11, "Primary Unit"=w472:T11)  [unwired: 6 in]
              n148 = call "LCR_AutoChangeUnits.vi"("Secondary Unit"=w471, "Primary Unit"=w472) -> ("Secondary Ref"=w469:refnum<vi>, "Primary Ref"=w470:refnum<vi>)  [unwired: 8 in]
            }
            frame "UpdatePlots" {
              n149 = control-ref of="Test Graph"() -> (w485:refnum<vi>)
              n150 = call "LCR_PlotHelper.vi"("Y-Axis"="Y-Axis", "X-Axis"="X-Axis", "Data_IN"=w482, "Graph REF"=w485) -> ("Graph Out"=→"Test Graph":cluster{"Variant X":dbl, "Variant Y":dbl}[], "Data_Out"=w481:T3)  [unwired: 6 in]
            }
            frame "RefreshPlotMUnits" {
              n151 = control-ref of="Test Graph"() -> (w492:refnum<vi>)
              n152 = property on="Y-Axis" class="Enum (strict)"() -> ("Value"=w490:T1)  [unwired: 2 in, 2 out]
              n153 = property on="X-Axis" class="Enum (strict)"() -> ("Value"=w491:T1)  [unwired: 2 in, 2 out]
              n154 = call "LCR_PlotNamer.vi"("Y-Axis"=w490, "X-Axis"=w491, "Graph Ref In"=w492) -> ("Secondary Ref"=w488:refnum<vi>, "Primary Ref"=w489:refnum<vi>)  [unwired: 7 in]
            }
            frame "ClearBuffers" {
              n155 = in-place {
                n156 = in-place-cluster #1(w500) -> ("Measurements"=w505:T4[])
                n157 = Array Size(array=w505) -> (size(s)=w504:i32)
                n158 = Delete From Array(array=w505, length=w504, index=0) -> (array with subset deleted=w507:T4[])  [unwired: 1 out]
                n159 = in-place-cluster #1("Measurements"=w507) -> (w499:T3)
              }
            }
          }
          n160 = Merge Errors(w33, w34) -> (w44:errorcluster)
          n161 = call "GEN_CulArray.vi"("Max Values"="Max Elements", "Data_Cluster"=w31) -> ("Data_Cluster Out"=w30:T3)  [unwired: 9 in]
          n162 = Or(x=w44, y=w43) -> (x .or. y?=w42:bool)
        }
      }
      frame Error {
      }
    }
  }
  n163 = while {
    tunnel: w8 -> [w512]
    tunnel: w9 -> [w511]
    tunnel: w6 -> [w509]
    stop <- w510 stop-if-true
    # "GUI Event Loop"
    n164 = event shown="[8] \"StopM_Button\": Value Change" {
      selector: _ -> [_ _ _ _ _ _ _ _ _ _ _ _ _ _]
      dyn-events: _ -> [_ _ _ _ _ _ _ _ _ _ _ _ _ _]
      timeout: _ -> [_ _ _ _ _ _ _ _ _ _ _ _ _ _]
      tunnel: w512 -> [_ w517 w522 w527 w532 w537 w542 w547 w552 w557 w562 w567 w572 w577]
      tunnel: w511 -> [_ w516 w521 w526 w531 w536 w541 w546 w551 w556 w561 w566 w571 w576]
      tunnel: [_ TRUE FALSE FALSE FALSE FALSE FALSE FALSE FALSE FALSE FALSE FALSE FALSE FALSE] -> w510
      tunnel: w509 -> [_ w513 w518 w523 w528 w533 w538 w543 w548 w553 w558 w563 w568 w573]
      event Timeout {
        n165 = event-data() -> ()  [unwired: 1 in, 3 out]
      }
      event "Exit_Button": Value Change {
        n166 = event-data() -> ()  [unwired: 1 in, 6 out]
        n167 = Set Occurrence(w513) -> ()
        n168 = Enqueue Element At Opposite End(queue=w517, element=cluster{T2, bool} {enum."ExitSafe", TRUE}, error in (no error)=w516) -> ()  [unwired: 1 in, 3 out]
      }
      event "Retry_Button": Value Change {
        n169 = event-data() -> ()  [unwired: 1 in, 6 out]
        n170 = Set Occurrence(w518) -> ()
        n171 = Enqueue Element At Opposite End(queue=w522, element=cluster{T2, bool} {enum."RetryComs", FALSE}, error in (no error)=w521) -> ()  [unwired: 1 in, 3 out]
      }
      event #3 (no event record) {
        n172 = event-data() -> ()  [unwired: 1 in, 6 out]
        n173 = Set Occurrence(w523) -> ()
        n174 = Enqueue Element(queue=w527, element=cluster{T12, bool} {enum."LoadProfile", FALSE}, error in (no error)=w526) -> ()  [unwired: 1 in, 3 out]
      }
      event "ApplyConfig_Button": Value Change {
        n175 = event-data() -> ()  [unwired: 1 in, 6 out]
        n176 = Set Occurrence(w528) -> ()
        n177 = Enqueue Element(queue=w532, element=cluster{T2, bool} {enum."Disconnect", FALSE}, error in (no error)=w531) -> ()  [unwired: 1 in, 3 out]
      }
      event #5 (no event record) {
        n178 = event-data() -> ()  [unwired: 1 in, 6 out]
        n179 = Set Occurrence(w533) -> ()
        n180 = Enqueue Element(queue=w537, element=cluster{T12, bool} {enum."SaveProfile", FALSE}, error in (no error)=w536) -> ()  [unwired: 1 in, 3 out]
      }
      event "SaveConfig_Button": Value Change {
        n181 = event-data() -> ()  [unwired: 1 in, 6 out]
        n182 = Set Occurrence(w538) -> ()
        n183 = Enqueue Element(queue=w542, element=cluster{T2, bool} {enum."SaveConfig", FALSE}, error in (no error)=w541) -> ()  [unwired: 1 in, 3 out]
      }
      event #7 (no event record) {
        n184 = event-data() -> ()  [unwired: 1 in, 6 out]
        n185 = Set Occurrence(w543) -> ()
        n186 = Enqueue Element(queue=w547, element=cluster{T2, bool} {enum."SendProfile", FALSE}, error in (no error)=w546) -> ()  [unwired: 1 in, 3 out]
      }
      event "StopM_Button": Value Change {
        n187 = event-data() -> ()  [unwired: 1 in, 6 out]
        n188 = Set Occurrence(w548) -> ()
        n189 = Enqueue Element(queue=w552, element=cluster{T2, bool} {enum."SwitchToOff", FALSE}, error in (no error)=w551) -> ()  [unwired: 1 in, 3 out]
      }
      event "Measure_Button": Value Change {
        n190 = event-data() -> ()  [unwired: 1 in, 6 out]
        n191 = Set Occurrence(w553) -> ()
        n192 = Enqueue Element(queue=w557, element=cluster{T2, bool} {enum."SwitchToMeas", FALSE}, error in (no error)=w556) -> ()  [unwired: 1 in, 3 out]
      }
      event "Log_Button": Value Change {
        n193 = event-data() -> ()  [unwired: 1 in, 6 out]
        n194 = Set Occurrence(w558) -> ()
        n195 = Enqueue Element(queue=w562, element=cluster{T2, bool} {enum."SwitchToLog", FALSE}, error in (no error)=w561) -> ()  [unwired: 1 in, 3 out]
      }
      event #11 (no event record) {
        n196 = event-data() -> ()  [unwired: 1 in, 6 out]
        n197 = Set Occurrence(w563) -> ()
        n198 = Enqueue Element(queue=w567, element=cluster{T2, bool} {enum."RefreshMUnits", FALSE}, error in (no error)=w566) -> ()  [unwired: 1 in, 3 out]
      }
      event "Clear_Button": Value Change {
        n199 = event-data() -> ()  [unwired: 1 in, 6 out]
        n200 = Set Occurrence(w568) -> ()
        n201 = Enqueue Element(queue=w572, element=cluster{T2, bool} {enum."ClearBuffers", FALSE}, error in (no error)=w571) -> ()  [unwired: 1 in, 3 out]
      }
      event Value Change {
        n202 = event-data() -> ()  [unwired: 1 in, 6 out]
        n203 = Set Occurrence(w573) -> ()
        n204 = Enqueue Element(queue=w577, element=cluster{T2, bool} {enum."RefreshPlotMUnits", FALSE}, error in (no error)=w576) -> ()  [unwired: 1 in, 3 out]
      }
    }
  }
  n205 = property on="Measuring" class="Bool (strict)"("Colors [4]"=w1) -> ()  [unwired: 2 in, 2 out]
  n206 = property on="Logging" class="Bool (strict)"("Colors [4]"=w1) -> ()  [unwired: 2 in, 2 out]
  "Globals" <- FALSE ("Globals")
  "AH 2500A" <- FALSE ("HM 8118")
  "Logging" <- FALSE ("Logging")
  "Measuring" <- FALSE ("Measuring")
